vi "ENPH 354 Assignment 1 - Q3.vi"() -> ()   [LabVIEW 2021]
panel:
  in  "y":i32
  out "2D Array":dbl[][](array[numeric])
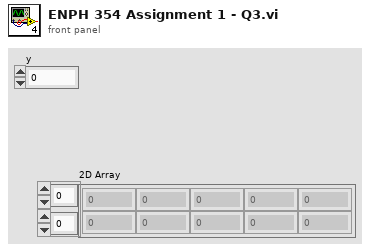
[diagram p1: front panel]
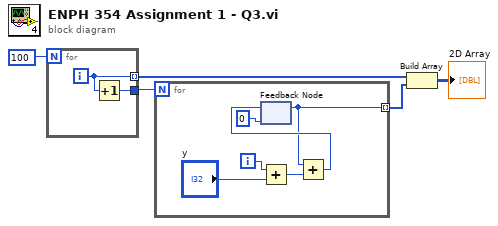
[diagram p0: block diagram]
diagram:
  n1 = for {
    N: 100 -> [_]
    tunnel: [w6] -> w4 mode=indexing
    tunnel: [w7] -> w1
    i -> [w6]
    n2 = Increment(x=w6) -> (x+1=w7:i32)
  }
  n3 = for {
    N: w1 -> [_]
    tunnel: [w12] -> w2 mode=indexing
    i -> [w10]
    n4 = feedback #1(0) -> (w12:i32)
    n5 = Add(x=w10, y="y") -> (x+y=w8:i32)
    n6 = Add(x=w12, y=w8) -> (x+y=w13:i32)
    n7 = feedback-in #1(w13) -> ()
  }
  n8 = Build Array(w4, w2) -> (→"2D Array":i32[][])
